vi "DSDLL Setup Virtual Channels.vi"(8 "error in":errorcluster, 9 "samples count":i32=48000, 10 "sample rate [Hz]":dbl=48000.0, 11 "dsdll session":T1) -> (0 "error out":errorcluster, 3 "dsdll session out":T1)   [LabVIEW 2020, in "DSDLL Virtual Digitizer.lvlib"]
doc: "Opens dsdll channels with given sampling rate."
uses:
  DSDLL Virtual Digitizer.lvlib
  DSDLL Session.ctl
  dsdll/dsdll_instance.ctl
  dsdll/dsdll_device_record.ctl
  DSDLL Process Config.ctl
  DSDLL Data Packet.ctl
  dsdll/dsdll_format.ctl
  dsdll/dsdll_sample_format.ctl
  <vilib>/Utility/error.llb/Error Cluster From Error Code.vi
  <vilib>/ErrorRing/Error Ring.xnode
  dsdll/dsdll.lvlib
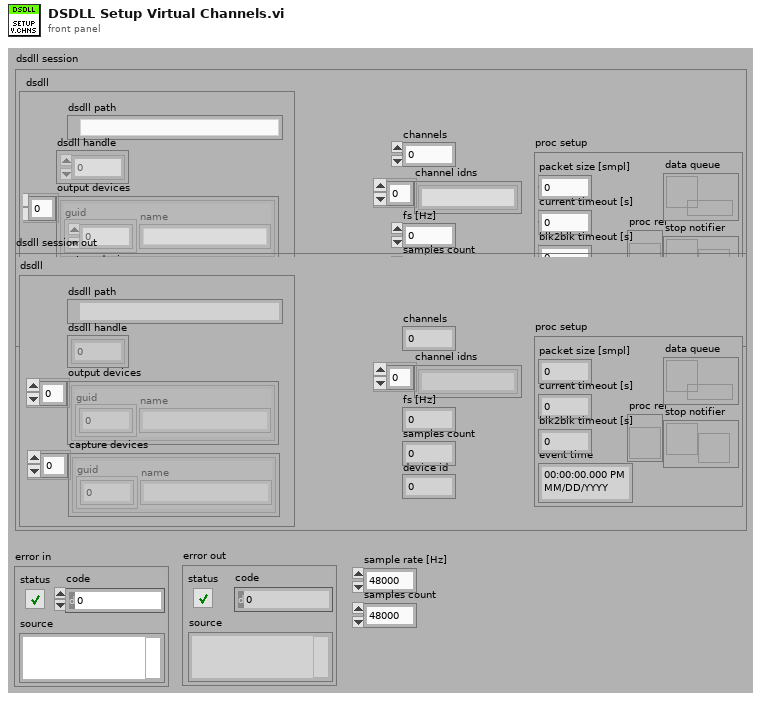
[diagram p1: front panel]
types:
  T1 = typedef "DSDLL Virtual Digitizer.lvlib/DSDLL Session.ctl" = cluster{"dsdll":T2, "channels":i32, "device id":i32, "channel idns":string[], "proc setup":T4, "samples count":i32, "fs [Hz]":dbl}
  T2 = typedef "dsdll.lvlib/dsdll_instance.ctl" = cluster{"dsdll path":path, "dsdll handle":u8[], "output devices":T3[], "capture devices":T3[]}
  T3 = typedef "dsdll.lvlib/dsdll_device_record.ctl" = cluster{"guid":u8[], "name":string}
  T4 = typedef "DSDLL Virtual Digitizer.lvlib/DSDLL Process Config.ctl" = cluster{"packet size [smpl]":i32, "current timeout [s]":dbl, "blk2blk timeout [s]":dbl, "event time":timestamp, "data queue":refnum<queue>, "stop notifier":refnum<notifier>, "proc ref":refnum<vi>}
  T5 = typedef "dsdll.lvlib/dsdll_sample_format.ctl" = enum16{"IEEE float 32", "PCM 16 bit"}
  T6 = typedef "dsdll.lvlib/dsdll_format.ctl" = cluster{"sample rate [Hz]":u32, "out channels":u16, "inp channels":u16, "format":T5}
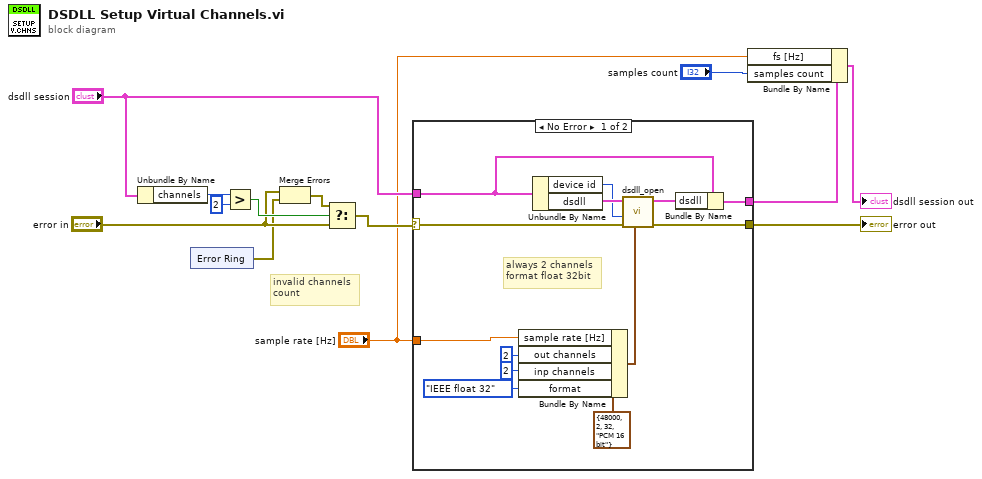
[diagram p0: block diagram]
diagram:
  # "invalid channels\ncount"
  n1 = Unbundle By Name("dsdll session") -> ("channels"=w13:i32)
  n2 = xnode "Error Ring"() -> ("error out"=w8:errorcluster)
  n3 = Greater?(x=w13, y=2) -> (0:w11:bool)
  n4 = Merge Errors("error in", w8) -> (w10:errorcluster)
  n5 = Select(t=w10, s=w11, f="error in") -> (s? t:f=w5:errorcluster)
  n6 = case shown="No Error" w5 {
    selector: w5 -> [w14 w28]
    tunnel: [w26 w27] -> w3
    tunnel: "sample rate [Hz]" -> [w18 _]
    tunnel: [w17 w28] -> w7
    tunnel: "dsdll session" -> [w15 w27]
    frame No Error {
      # "always 2 channels\nformat float 32bit"
      n7 = Bundle By Name(cluster=T6 {"sample rate [Hz]"=48000, "out channels"=2, "inp channels"=32, "format"=enum."PCM 16 bit"} ("format"), "sample rate [Hz]"=w18, "out channels"=u16 2, "inp channels"=u16 2, "format"=dsdll_sample_format."IEEE float 32") -> (w23:T6)
      n8 = Unbundle By Name(w15) -> ("device id"=w24:i32, "dsdll"=w25:T2)
      n9 = call "dsdll_open.vi"("format"=w23, "error in"=w14, "capture device id"=w24, "dsdll instance in"=w25) -> ("error out"=w17:errorcluster, "dsdll instance out"=w16:T2)  [unwired: 6 in]
      n10 = Bundle By Name(cluster=w15, "dsdll"=w16) -> (w26:T1)
    }
    frame Error {
    }
  }
  "error out" <- w7
  n11 = Bundle By Name(cluster=w3, "fs [Hz]"="sample rate [Hz]", "samples count"="samples count") -> (→"dsdll session out":T1)
